vi "UDP Begin Test.vi"() -> ()   [LabVIEW 2014, in "ESP8266 WiFi Wrapper.lvlib"]
uses:
  <vilib>/Aledyne-TSXperts/Arduino Compatible Compiler for LabVIEW/addons/ESP8266 WiFi Wrapper/ESP8266 WiFi Wrapper.lvlib
panel:
  out "Is listening?":bool
  in  "Port":i16
  out "Error Out":errorcluster
  in  "Error In":errorcluster
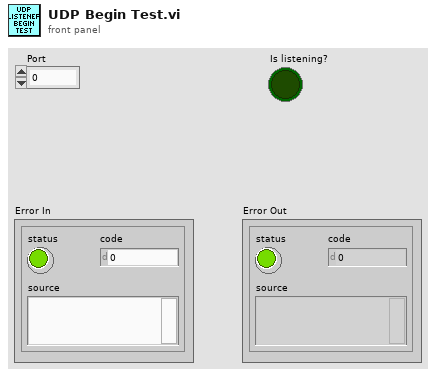
[diagram p1: front panel]
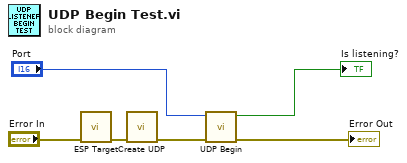
[diagram p0: block diagram]
diagram:
  n1 = call <vilib>:"ESP Target.vi"("Error In"="Error In") -> ("Error Out"=w1:errorcluster)  [unwired: 10 in]
  n2 = call <vilib>:"Create UDP.vi"("Error In"=w1) -> ("Error Out"=w3:errorcluster)  [unwired: 10 in]
  n3 = call <vilib>:"UDP Begin.vi"("Error In"=w3, "Port"="Port") -> ("Error Out"=→"Error Out":errorcluster, "Is listening?"=→"Is listening?":bool)  [unwired: 8 in]
